vi "FTW-JSON-Core-GetFlattenedValue.vi"(0 "JSON Element":i64 format="%016x", 5 "Element Data Name":string, 7 "LabVIEW Type":T1, 9 "Element Default Value":variant, 11 "error in":errorcluster) -> (4 "Flattened Value":string, 15 "error out":errorcluster)   [LabVIEW 2012]
uses:
  Reflection/FTW-Reflection-Types.ctl
  FTW-JSON-Type.ctl
panel:
  # "Inputs"
  # "Outputs"
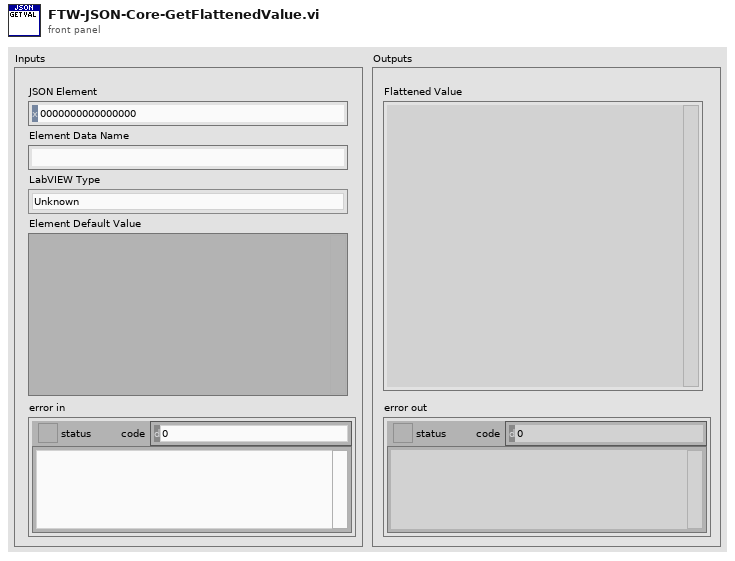
[diagram p1: front panel]
types:
  T1 = typedef "FTW-Reflection-Types.ctl" = enum16{"Unknown", "Void", "Array", "Cluster", "LVObject", "Boolean", "I8", "I16", "I32", "I64", "U8", "U16", "U32", "U64", "SGL", "DBL", "EXT", "CSG", "CDB", "CXT", "FXP", "EnumU8", "EnumU16", "EnumU32", "EnumU64", "SGLwithUnit", "DBLwithUnit", "EXTwithUnit", "CSGwithUnit", "CDBwithUnit", "CXTwithUnit", "String", "Path", "Picture", "Tag", "LVVariant", "Timestamp", "WaveformI8", "WaveformI16", "WaveformI32", "WaveformI64", "WaveformU8", "WaveformU16", "WaveformU32", "WaveformU64", "WaveformSGL", "WaveformDBL", "WaveformEXT", "WaveformCSG", "WaveformCDB", "WaveformCXT", "WaveformDigital", "WaveformUnknownType", "DigitalData", "DynamicData", "ExternalData", "FileByteStream", "TDMStream", "dotNET", "ActiveX", "VIServerReference", "VIReference", "ApplicationInstance", "Menu", "ConnectionDataSocket", "ConnectionVISA", "ConnectionBluetooth", "ConnectionIrDA", "ConnectionTCP", "ConnectionUDP", "ConnectionHTTPClient", "ConnectionFTP", "Occurrence", "Notifier", "Queue", "Rendezvous", "Semaphore", "RTFIFO", "EventPublisher", "EventRegistration", "EventCallback", "DataValueReference", "GenericClass", "GenericClassTag", "GenericClassDeepCopy", "GenericClassFlattened", "GenericClassTagFlattened", "GenericReferenceType", "WindowsRegistry", "OverloadedDatalogRef", "ReferenceUnknownType"}
  T2 = typedef "FTW-JSON-Type.ctl" = enum16{"Object", "Array", "String", "Integer", "Floating Point", "true", "false", "null", "undefined"}
  T3 = cluster{"Element Name":string, "Element Type":T1, "Element Value":variant}[]
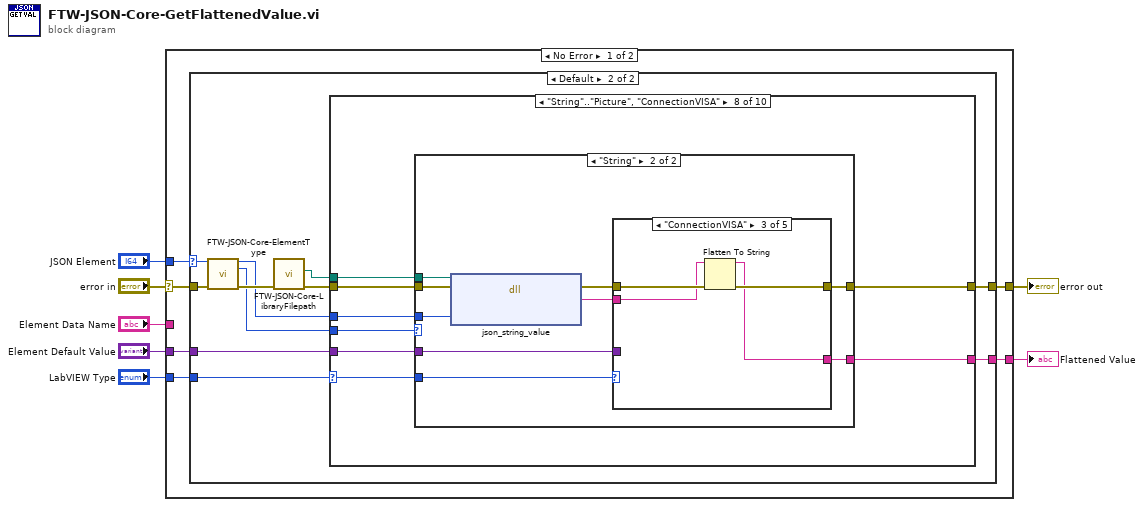
[diagram p0: block diagram]
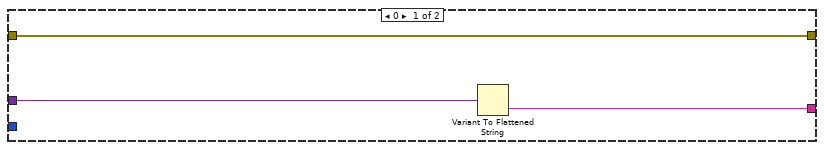
[diagram p2: hidden frame]
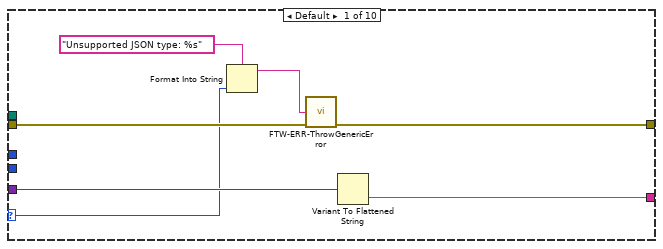
[diagram p3: hidden frame]
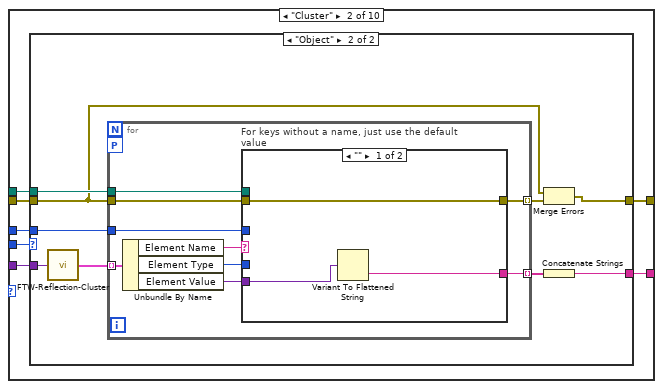
[diagram p4: hidden frame]
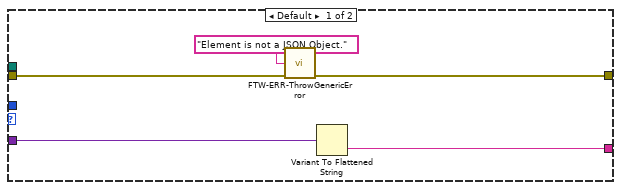
[diagram p5: hidden frame]
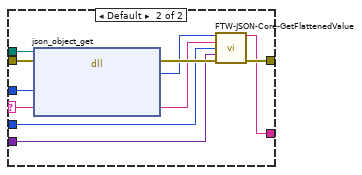
[diagram p6: hidden frame]
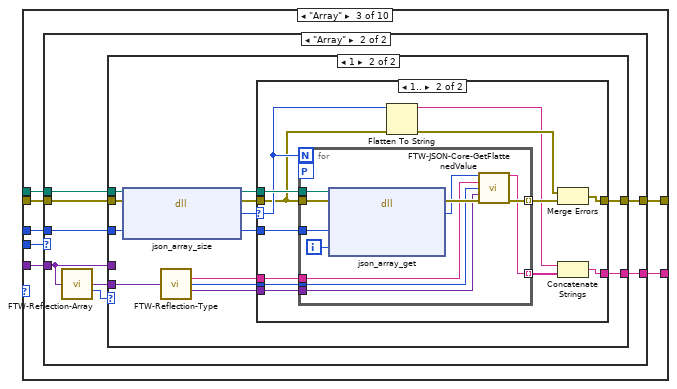
[diagram p7: hidden frame]
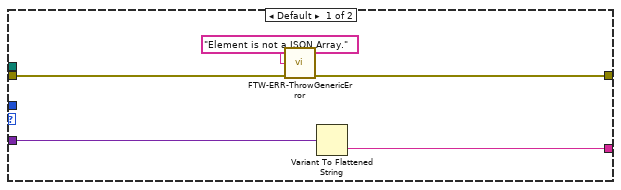
[diagram p8: hidden frame]
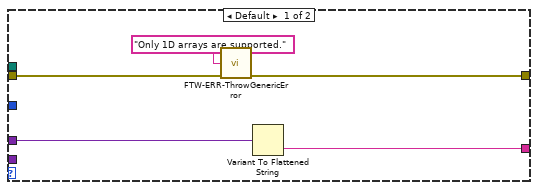
[diagram p9: hidden frame]
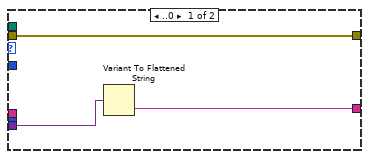
[diagram p10: hidden frame]
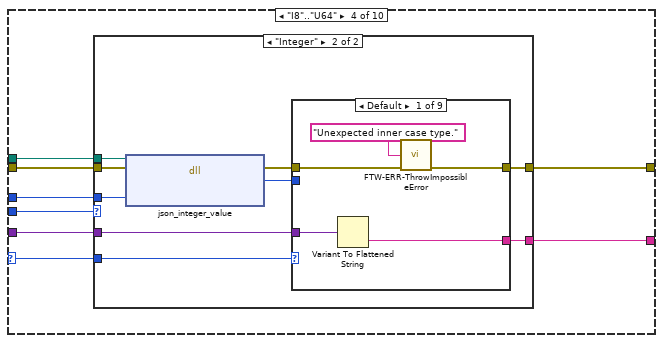
[diagram p11: hidden frame]
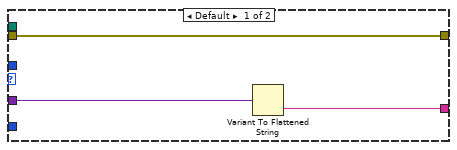
[diagram p12: hidden frame]
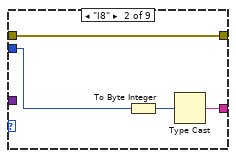
[diagram p13: hidden frame]
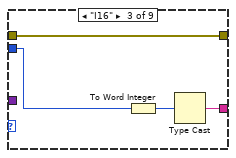
[diagram p14: hidden frame]
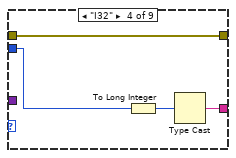
[diagram p15: hidden frame]
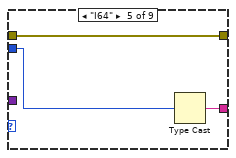
[diagram p16: hidden frame]
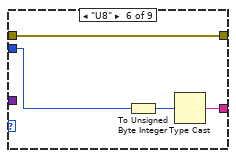
[diagram p17: hidden frame]
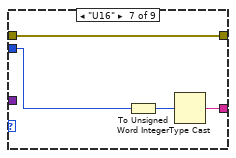
[diagram p18: hidden frame]
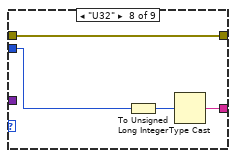
[diagram p19: hidden frame]
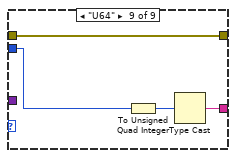
[diagram p20: hidden frame]
diagram:
  n1 = case shown="No Error" "error in" {
    selector: "error in" -> [w9 w424]
    tunnel: [w13 w424] -> w7
    tunnel: "JSON Element" -> [w8 _]
    tunnel: [w12 w422] -> w5
    tunnel: "LabVIEW Type" -> [w11 _]
    tunnel: "Element Default Value" -> [w10 w423]
    tunnel: "Element Data Name" -> [_ _]
    frame No Error {
      n2 = case shown="Default" w8 {
        selector: w8 -> [_ w17]
        tunnel: [w14 w27] -> w13
        tunnel: [w15 w26] -> w12
        tunnel: w11 -> [_ w23]
        tunnel: w10 -> [w16 w22]
        tunnel: w9 -> [w14 w21]
        frame 0 {
          n3 = Variant To Flattened String(Variant=w16) -> (data string=w15:string)  [unwired: 1 out]
        }
        frame Default {
          n4 = call "FTW-JSON-Core-ElementType.vi"("JSON Element"=w17, "error in"=w21) -> ("JSON Element out"=w19:i64, "JSON Type"=w18:T2, "error out"=w20:errorcluster)  [unwired: 11 in]
          n5 = call "FTW-JSON-Core-LibraryFilepath.vi"("error in"=w20) -> ("error out"=w25:errorcluster, "JSON Library Filepath"=w24:path)  [unwired: 9 in]
          n6 = case shown="\"String\"..\"Picture\", \"ConnectionVISA\"" w23 {
            selector: w23 -> [w28 _ _ w147 w203 w286 _ w339 _ _]
            tunnel: [w31 w37 w83 w144 w200 w283 w319 w336 w378 w409] -> w27
            tunnel: [w29 w40 w84 w149 w205 w288 w323 w341 w382 w412] -> w26
            tunnel: w25 -> [w32 w36 w82 w150 w206 w289 w324 w342 w383 w413]
            tunnel: w24 -> [_ w39 w80 w151 w207 w290 w325 w343 w384 _]
            tunnel: w19 -> [_ w38 w79 w146 w202 w285 w321 w338 w380 _]
            tunnel: w22 -> [w30 w41 w85 w148 w204 w287 w322 w340 w381 w411]
            tunnel: w18 -> [_ w35 w81 w145 w201 w284 w320 w337 w379 w410]
            frame Default {
              n7 = Format Into String(format string="Unsupported JSON type: %s", w28) -> (resulting string=w34:string)  [unwired: 2 in, 1 out]
              n8 = call "FTW-ERR-ThrowGenericError.vi"("Error Message"=w34, "error in"=w32) -> ("error out"=w31:errorcluster)  [unwired: 13 in]
              n9 = Variant To Flattened String(Variant=w30) -> (data string=w29:string)  [unwired: 1 out]
            }
            frame "Cluster" {
              n10 = case shown="\"Object\"" w35 {
                tunnel: w41 -> [w44 w54]
                tunnel: [w43 w52] -> w40
                tunnel: w39 -> [_ w51]
                tunnel: w38 -> [_ w49]
                tunnel: [w45 w48] -> w37
                tunnel: w36 -> [w46 w47]
                frame Default {
                  n11 = call "FTW-ERR-ThrowGenericError.vi"("Error Message"="Element is not a JSON Object.", "error in"=w46) -> ("error out"=w45:errorcluster)  [unwired: 13 in]
                  n12 = Variant To Flattened String(Variant=w44) -> (data string=w43:string)  [unwired: 1 out]
                }
                frame "Object" {
                  n13 = call "FTW-Reflection-Cluster.vi"("Cluster"=w54) -> ("Cluster Elements"=w55:T3)  [unwired: 14 in]
                  n14 = for {
                    tunnel: w55 -> [w63] mode=indexing
                    tunnel: [w60] -> w53 mode=indexing
                    tunnel: w51 -> [w57]
                    tunnel: w49 -> [w56]
                    tunnel: w47 -> [w64]
                    tunnel: [w58] -> w50 mode=indexing
                    workers-P: _ -> [_]
                    n15 = Unbundle By Name(w63) -> ("Element Name"=w62:string, "Element Type"=w59:T1, "Element Value"=w61:variant)
                    n16 = case "For keys without a name, just use the default value" shown="\"\"" w62 {
                      selector: w62 -> [_ w74]
                      tunnel: w57 -> [_ w77]
                      tunnel: w64 -> [w65 w76]
                      tunnel: w61 -> [w67 w70]
                      tunnel: [w66 w71] -> w60
                      tunnel: w56 -> [_ w75]
                      tunnel: w59 -> [_ w69]
                      tunnel: [w65 w72] -> w58
                      frame "" {
                        n17 = Variant To Flattened String(Variant=w67) -> (data string=w66:string)  [unwired: 1 out]
                      }
                      frame Default {
                        n18 = dll-call lib="?" fn="json_object_get"(path in=w77, error in=w76, "JSON Object Pointer"=w75, "Element Key"=w74) -> (error out=w78:errorcluster, "JSON Element Pointer"=w73:i64, "Element Key"=w68:string)  [unwired: 2 in, 1 out]
                        n19 = call "FTW-JSON-Core-GetFlattenedValue.vi"("JSON Element"=w73, "Element Data Name"=w68, "LabVIEW Type"=w69, "Element Default Value"=w70, "error in"=w78) -> ("Flattened Value"=w71:string, "error out"=w72:errorcluster)  [unwired: 9 in]
                      }
                    }
                  }
                  n20 = Merge Errors(w47, w50) -> (w48:errorcluster)
                  n21 = Concatenate Strings(w53) -> (w52:string)
                }
              }
            }
            frame "Array" {
              n22 = case shown="\"Array\"" w81 {
                tunnel: w85 -> [w88 w91]
                tunnel: [w87 w98] -> w84
                tunnel: [w86 w97] -> w83
                tunnel: w82 -> [w89 w96]
                tunnel: w80 -> [_ w93]
                tunnel: w79 -> [_ w92]
                frame Default {
                  n23 = call "FTW-ERR-ThrowGenericError.vi"("Error Message"="Element is not a JSON Array.", "error in"=w89) -> ("error out"=w86:errorcluster)  [unwired: 13 in]
                  n24 = Variant To Flattened String(Variant=w88) -> (data string=w87:string)  [unwired: 1 out]
                }
                frame "Array" {
                  n25 = call "FTW-Reflection-Array.vi"("Array"=w91) -> ("Default Array Element"=w95:variant, "Number of Dimensions"=w94:i32)  [unwired: 13 in]
                  n26 = case shown="1" w94 {
                    tunnel: [w100 w116] -> w98
                    tunnel: [w101 w115] -> w97
                    tunnel: w96 -> [w102 w114]
                    tunnel: w95 -> [_ w108]
                    tunnel: w93 -> [_ w113]
                    tunnel: w92 -> [_ w112]
                    tunnel: w91 -> [w99 _]
                    frame Default {
                      n27 = call "FTW-ERR-ThrowGenericError.vi"("Error Message"="Only 1D arrays are supported.", "error in"=w102) -> ("error out"=w101:errorcluster)  [unwired: 13 in]
                      n28 = Variant To Flattened String(Variant=w99) -> (data string=w100:string)  [unwired: 1 out]
                    }
                    frame 1 {
                      n29 = dll-call lib="?" fn="json_array_size"(path in=w113, error in=w114, "Array Pointer"=w112) -> (path out=w111:path, error out=w109:errorcluster, "Array Size"=w105:i32, "Array Pointer"=w110:i64)  [unwired: 1 in]
                      n30 = call "FTW-Reflection-Type.vi"("Anything"=w108) -> ("Data Name"=w104:string, "LabVIEW Type"=w107:T1, "Variant Type and Value"=w106:variant)  [unwired: 12 in]
                      n31 = case shown="1.." w105 {
                        selector: w105 -> [_ w124]
                        tunnel: [w119 w132] -> w116
                        tunnel: [w117 w131] -> w115
                        tunnel: w111 -> [_ w130]
                        tunnel: w110 -> [_ w129]
                        tunnel: w109 -> [w117 w121]
                        tunnel: w107 -> [_ w127]
                        tunnel: w106 -> [w118 w126]
                        tunnel: w104 -> [_ w120]
                        frame ..0 {
                          n32 = Variant To Flattened String(Variant=w118) -> (data string=w119:string)  [unwired: 1 out]
                        }
                        frame 1.. {
                          n33 = for {
                            N: w124 -> [_]
                            tunnel: w130 -> [w142]
                            tunnel: w129 -> [w140]
                            workers-P: _ -> [_]
                            tunnel: w121 -> [w141]
                            tunnel: [w138] -> w128 mode=indexing
                            tunnel: w127 -> [w134]
                            tunnel: w126 -> [w135]
                            tunnel: [w136] -> w125 mode=indexing
                            tunnel: w120 -> [w133]
                            i -> [w139]
                            n34 = dll-call lib="?" fn="json_array_get"(path in=w142, error in=w141, "Array Pointer"=w140, "Index"=w139) -> (error out=w143:errorcluster, "Array Element"=w137:i64)  [unwired: 3 in, 1 out]
                            n35 = call "FTW-JSON-Core-GetFlattenedValue.vi"("JSON Element"=w137, "Element Data Name"=w133, "LabVIEW Type"=w134, "Element Default Value"=w135, "error in"=w143) -> ("Flattened Value"=w136:string, "error out"=w138:errorcluster)  [unwired: 9 in]
                          }
                          n36 = Flatten To String(anything=w124, error in (no error)=w121) -> (data string=w122:string, error out=w123:errorcluster)  [unwired: 2 in, 1 out]
                          n37 = Merge Errors(w123, w128) -> (w131:errorcluster)
                          n38 = Concatenate Strings(w122, w125) -> (w132:string)
                        }
                      }
                    }
                  }
                }
              }
            }
            frame "I8".."U64" {
              n39 = case shown="\"Integer\"" w145 {
                tunnel: w151 -> [_ w163]
                tunnel: w146 -> [_ w162]
                tunnel: w150 -> [w152 w161]
                tunnel: w148 -> [w154 w155]
                tunnel: [w153 w156] -> w149
                tunnel: [w152 w159] -> w144
                tunnel: w147 -> [_ w160]
                frame Default {
                  n40 = Variant To Flattened String(Variant=w154) -> (data string=w153:string)  [unwired: 1 out]
                }
                frame "Integer" {
                  n41 = dll-call lib="?" fn="json_integer_value"(path in=w163, error in=w161, "JSON Element Pointer"=w162) -> (error out=w158:errorcluster, "I64 Value"=w157:i64)  [unwired: 2 in, 1 out]
                  n42 = case shown="Default" w160 {
                    tunnel: [w167 w172 w176 w180 w183 w187 w191 w195 w199] -> w159
                    tunnel: w158 -> [w168 w172 w176 w180 w183 w187 w191 w195 w199]
                    tunnel: w157 -> [_ w170 w174 w178 w181 w185 w189 w193 w197]
                    tunnel: [w164 w171 w175 w179 w182 w186 w190 w194 w198] -> w156
                    tunnel: w155 -> [w165 _ _ _ _ _ _ _ _]
                    frame Default {
                      n43 = Variant To Flattened String(Variant=w165) -> (data string=w164:string)  [unwired: 1 out]
                      n44 = call "FTW-ERR-ThrowImpossibleError.vi"("Reason this error should never happen"="Unexpected inner case type.", "error in"=w168) -> ("error out"=w167:errorcluster)  [unwired: 13 in]
                    }
                    frame "I8" {
                      n45 = To Byte Integer(number=w170) -> (8bit integer=w169:i8)
                      n46 = Type Cast(x=w169) -> (*(type *) &x=w171:string)  [unwired: 1 in]
                    }
                    frame "I16" {
                      n47 = To Word Integer(number=w174) -> (16bit integer=w173:i16)
                      n48 = Type Cast(x=w173) -> (*(type *) &x=w175:string)  [unwired: 1 in]
                    }
                    frame "I32" {
                      n49 = To Long Integer(number=w178) -> (32bit integer=w177:i32)
                      n50 = Type Cast(x=w177) -> (*(type *) &x=w179:string)  [unwired: 1 in]
                    }
                    frame "I64" {
                      n51 = Type Cast(x=w181) -> (*(type *) &x=w182:string)  [unwired: 1 in]
                    }
                    frame "U8" {
                      n52 = To Unsigned Byte Integer(number=w185) -> (unsigned 8bit integer=w184:u8)
                      n53 = Type Cast(x=w184) -> (*(type *) &x=w186:string)  [unwired: 1 in]
                    }
                    frame "U16" {
                      n54 = To Unsigned Word Integer(number=w189) -> (unsigned 16bit integer=w188:u16)
                      n55 = Type Cast(x=w188) -> (*(type *) &x=w190:string)  [unwired: 1 in]
                    }
                    frame "U32" {
                      n56 = To Unsigned Long Integer(number=w193) -> (unsigned 32bit integer=w192:u32)
                      n57 = Type Cast(x=w192) -> (*(type *) &x=w194:string)  [unwired: 1 in]
                    }
                    frame "U64" {
                      n58 = To Unsigned Quad Integer(1:w197) -> (0:w196:u64)
                      n59 = Type Cast(x=w196) -> (*(type *) &x=w198:string)  [unwired: 1 in]
                    }
                  }
                }
              }
            }
            frame "EnumU8".."EnumU64" {
              n60 = case shown="\"Integer\"" w201 {
                tunnel: w207 -> [_ w219 w259]
                tunnel: w202 -> [_ w218 w257]
                tunnel: w206 -> [w208 w217 w258]
                tunnel: w204 -> [w210 w211 w256]
                tunnel: [w209 w212 w253] -> w205
                tunnel: [w208 w215 w254] -> w200
                tunnel: w203 -> [_ w216 w255]
                frame Default {
                  n61 = Variant To Flattened String(Variant=w210) -> (data string=w209:string)  [unwired: 1 out]
                }
                frame "String" {
                  n62 = dll-call lib="?" fn="json_string_value"(path in=w219, error in=w217, "JSON Element Pointer"=w218) -> (error out=w214:errorcluster, "String Value"=w213:string)  [unwired: 2 in, 1 out]
                  n63 = case shown="Default" w216 {
                    tunnel: [w223 w231 w238 w245 w252] -> w215
                    tunnel: w214 -> [w224 w231 w238 w245 w252]
                    tunnel: w213 -> [_ w228 w235 w242 w249]
                    tunnel: [w220 w227 w234 w241 w248] -> w212
                    tunnel: w211 -> [w221 w230 w237 w244 w251]
                    frame Default {
                      n64 = Variant To Flattened String(Variant=w221) -> (data string=w220:string)  [unwired: 1 out]
                      n65 = call "FTW-ERR-ThrowImpossibleError.vi"("Reason this error should never happen"="Unexpected inner case type.", "error in"=w224) -> ("error out"=w223:errorcluster)  [unwired: 13 in]
                    }
                    frame "EnumU8" {
                      n66 = call "FTW-Reflection-Enum.vi"("Enum"=w230) -> ("Enum Items"=w229:string[])  [unwired: 12 in, 2 out]
                      n67 = Search 1D Array(1D array=w229, element=w228) -> (index of element=w226:i32)  [unwired: 1 in]
                      n68 = To Unsigned Byte Integer(number=w226) -> (unsigned 8bit integer=w225:u8)
                      n69 = Type Cast(x=w225) -> (*(type *) &x=w227:string)  [unwired: 1 in]
                    }
                    frame "EnumU16" {
                      n70 = call "FTW-Reflection-Enum.vi"("Enum"=w237) -> ("Enum Items"=w236:string[])  [unwired: 12 in, 2 out]
                      n71 = Search 1D Array(1D array=w236, element=w235) -> (index of element=w233:i32)  [unwired: 1 in]
                      n72 = To Unsigned Word Integer(number=w233) -> (unsigned 16bit integer=w232:u16)
                      n73 = Type Cast(x=w232) -> (*(type *) &x=w234:string)  [unwired: 1 in]
                    }
                    frame "EnumU32" {
                      n74 = call "FTW-Reflection-Enum.vi"("Enum"=w244) -> ("Enum Items"=w243:string[])  [unwired: 12 in, 2 out]
                      n75 = Search 1D Array(1D array=w243, element=w242) -> (index of element=w240:i32)  [unwired: 1 in]
                      n76 = To Unsigned Long Integer(number=w240) -> (unsigned 32bit integer=w239:u32)
                      n77 = Type Cast(x=w239) -> (*(type *) &x=w241:string)  [unwired: 1 in]
                    }
                    frame "EnumU64" {
                      n78 = call "FTW-Reflection-Enum.vi"("Enum"=w251) -> ("Enum Items"=w250:string[])  [unwired: 12 in, 2 out]
                      n79 = Search 1D Array(1D array=w250, element=w249) -> (index of element=w247:i32)  [unwired: 1 in]
                      n80 = To Unsigned Quad Integer(1:w247) -> (0:w246:u64)
                      n81 = Type Cast(x=w246) -> (*(type *) &x=w248:string)  [unwired: 1 in]
                    }
                  }
                }
                frame "Integer" {
                  n82 = dll-call lib="?" fn="json_integer_value"(path in=w259, error in=w258, "JSON Element Pointer"=w257) -> (error out=w261:errorcluster, "I64 Value"=w260:i64)  [unwired: 2 in, 1 out]
                  n83 = case shown="Default" w255 {
                    tunnel: [w265 w270 w274 w278 w282] -> w254
                    tunnel: w261 -> [w266 w270 w274 w278 w282]
                    tunnel: w260 -> [_ w268 w272 w276 w280]
                    tunnel: [w262 w269 w273 w277 w281] -> w253
                    tunnel: w256 -> [w263 _ _ _ _]
                    frame Default {
                      n84 = Variant To Flattened String(Variant=w263) -> (data string=w262:string)  [unwired: 1 out]
                      n85 = call "FTW-ERR-ThrowImpossibleError.vi"("Reason this error should never happen"="Unexpected inner case type.", "error in"=w266) -> ("error out"=w265:errorcluster)  [unwired: 13 in]
                    }
                    frame "EnumU8" {
                      n86 = To Unsigned Byte Integer(number=w268) -> (unsigned 8bit integer=w267:u8)
                      n87 = Type Cast(x=w267) -> (*(type *) &x=w269:string)  [unwired: 1 in]
                    }
                    frame "EnumU16" {
                      n88 = To Unsigned Word Integer(number=w272) -> (unsigned 16bit integer=w271:u16)
                      n89 = Type Cast(x=w271) -> (*(type *) &x=w273:string)  [unwired: 1 in]
                    }
                    frame "EnumU32" {
                      n90 = To Unsigned Long Integer(number=w276) -> (unsigned 32bit integer=w275:u32)
                      n91 = Type Cast(x=w275) -> (*(type *) &x=w277:string)  [unwired: 1 in]
                    }
                    frame "EnumU64" {
                      n92 = To Unsigned Quad Integer(1:w280) -> (0:w279:u64)
                      n93 = Type Cast(x=w279) -> (*(type *) &x=w281:string)  [unwired: 1 in]
                    }
                  }
                }
              }
            }
            frame "SGL".."EXT" {
              n94 = case shown="\"Integer\", \"Floating Point\"" w284 {
                tunnel: w290 -> [_ w302]
                tunnel: w285 -> [_ w301]
                tunnel: w289 -> [w291 w300]
                tunnel: w287 -> [w293 w294]
                tunnel: [w292 w295] -> w288
                tunnel: [w291 w298] -> w283
                tunnel: w286 -> [_ w299]
                frame Default {
                  n95 = Variant To Flattened String(Variant=w293) -> (data string=w292:string)  [unwired: 1 out]
                }
                frame "Integer", "Floating Point" {
                  n96 = dll-call lib="?" fn="json_number_value"(path in=w302, error in=w300, "JSON Element Pointer"=w301) -> (error out=w297:errorcluster, "DBL Value"=w296:dbl)  [unwired: 2 in, 1 out]
                  n97 = case shown="Default" w299 {
                    tunnel: [w306 w311 w314 w318] -> w298
                    tunnel: w297 -> [w307 w311 w314 w318]
                    tunnel: w296 -> [_ w308 w312 w316]
                    tunnel: [w303 w310 w313 w317] -> w295
                    tunnel: w294 -> [w304 _ _ _]
                    frame Default {
                      n98 = Variant To Flattened String(Variant=w304) -> (data string=w303:string)  [unwired: 1 out]
                      n99 = call "FTW-ERR-ThrowImpossibleError.vi"("Reason this error should never happen"="Unexpected inner case type.", "error in"=w307) -> ("error out"=w306:errorcluster)  [unwired: 13 in]
                    }
                    frame "SGL" {
                      n100 = To Single Precision Float(number=w308) -> (single precision float=w309:sgl)
                      n101 = Type Cast(x=w309) -> (*(type *) &x=w310:string)  [unwired: 1 in]
                    }
                    frame "DBL" {
                      n102 = Type Cast(x=w312) -> (*(type *) &x=w313:string)  [unwired: 1 in]
                    }
                    frame "EXT" {
                      n103 = To Extended Precision Float(1:w316) -> (0:w315:ext)
                      n104 = Type Cast(x=w315) -> (*(type *) &x=w317:string)  [unwired: 1 in]
                    }
                  }
                }
              }
            }
            frame "Timestamp" {
              n105 = case shown="Default" w320 {
                tunnel: w325 -> [_ w335]
                tunnel: w321 -> [_ w334]
                tunnel: w324 -> [w326 w333]
                tunnel: w322 -> [w328 _]
                tunnel: [w327 w331] -> w323
                tunnel: [w326 w332] -> w319
                frame Default {
                  n106 = Variant To Flattened String(Variant=w328) -> (data string=w327:string)  [unwired: 1 out]
                }
                frame "Floating Point" {
                  n107 = dll-call lib="?" fn="json_number_value"(path in=w335, error in=w333, "JSON Element Pointer"=w334) -> (error out=w332:errorcluster, "DBL Value"=w330:dbl)  [unwired: 2 in, 1 out]
                  n108 = To Time Stamp(1:w330) -> (0:w329:timestamp)
                  n109 = Type Cast(x=w329) -> (*(type *) &x=w331:string)  [unwired: 1 in]
                }
              }
            }
            frame "String".."Picture", "ConnectionVISA" {
              n110 = case shown="\"String\"" w337 {
                tunnel: w343 -> [_ w355]
                tunnel: w338 -> [_ w354]
                tunnel: w342 -> [w344 w353]
                tunnel: w340 -> [w346 w347]
                tunnel: [w345 w348] -> w341
                tunnel: [w344 w351] -> w336
                tunnel: w339 -> [_ w352]
                frame Default {
                  n111 = Variant To Flattened String(Variant=w346) -> (data string=w345:string)  [unwired: 1 out]
                }
                frame "String" {
                  n112 = dll-call lib="?" fn="json_string_value"(path in=w355, error in=w353, "JSON Element Pointer"=w354) -> (error out=w350:errorcluster, "String Value"=w349:string)  [unwired: 2 in, 1 out]
                  n113 = case shown="\"ConnectionVISA\"" w352 {
                    tunnel: [w359 w363 w367 w372 w377] -> w351
                    tunnel: w350 -> [w360 w364 w368 w373 w377]
                    tunnel: w349 -> [_ w362 w366 w371 w376]
                    tunnel: [w356 w361 w365 w370 w375] -> w348
                    tunnel: w347 -> [w357 _ _ _ _]
                    frame Default {
                      n114 = Variant To Flattened String(Variant=w357) -> (data string=w356:string)  [unwired: 1 out]
                      n115 = call "FTW-ERR-ThrowImpossibleError.vi"("Reason this error should never happen"="Unexpected inner case type.", "error in"=w360) -> ("error out"=w359:errorcluster)  [unwired: 13 in]
                    }
                    frame "String" {
                      n116 = Flatten To String(anything=w362, error in (no error)=w364) -> (data string=w361:string, error out=w363:errorcluster)  [unwired: 2 in, 1 out]
                    }
                    frame "ConnectionVISA" {
                      n117 = Flatten To String(anything=w366, error in (no error)=w368) -> (data string=w365:string, error out=w367:errorcluster)  [unwired: 2 in, 1 out]
                    }
                    frame "Path" {
                      n118 = String To Path(string=w371) -> (path=w369:path)
                      n119 = Flatten To String(anything=w369, error in (no error)=w373) -> (data string=w370:string, error out=w372:errorcluster)  [unwired: 2 in, 1 out]
                    }
                    frame "Picture" {
                      n120 = call "FTW-STR-Encode-Base64.vi"("Input"=w376, "Direction"=enum16{"Encode", "Decode"}."Decode") -> ("Output"=w375:string)
                    }
                  }
                }
              }
            }
            frame "FileByteStream".."ConnectionDataSocket", "ConnectionBluetooth".."ReferenceUnknownType" {
              n121 = case shown="\"String\"" w379 {
                tunnel: w384 -> [_ w399]
                tunnel: w380 -> [_ w398]
                tunnel: w383 -> [w385 w397]
                tunnel: w381 -> [w387 w392]
                tunnel: [w386 w394] -> w382
                tunnel: [w385 w390] -> w378
                frame Default {
                  n122 = Variant To Flattened String(Variant=w387) -> (data string=w386:string)  [unwired: 1 out]
                }
                frame "String" {
                  w395 = "0x%16x"  # Reference Format
                  n123 = dll-call lib="?" fn="json_string_value"(path in=w399, error in=w397, "JSON Element Pointer"=w398) -> (error out=w389:errorcluster, "String Value"=w396:string, "JSON Element Pointer"=w388:i64)  [unwired: 1 in, 1 out]
                  n124 = Scan From String(format string=w395, input string=w396, error in=w389, default 1=w388) -> (error out=w391:errorcluster, output 1=w393:i64)  [unwired: 1 in, 2 out]
                  n125 = case shown="No Error" w391 {
                    selector: w391 -> [w400 _]
                    tunnel: [w404 w407] -> w394
                    tunnel: w393 -> [w403 _]
                    tunnel: w392 -> [_ w408]
                    tunnel: [w400 w406] -> w390
                    frame No Error {
                      n126 = Type Cast(type=refnum<k0> refnum, x=w403) -> (*(type *) &x=w402:refnum<k0>)
                      n127 = Type Cast(x=w402) -> (*(type *) &x=w404:string)  [unwired: 1 in]
                    }
                    frame Error {
                      n128 = Variant To Flattened String(Variant=w408) -> (data string=w407:string)  [unwired: 1 out]
                      n129 = call "FTW-ERR-ThrowGenericError.vi"("Error Message"="Unexpected reference format.") -> ("error out"=w406:errorcluster)  [unwired: 14 in]
                    }
                  }
                }
              }
            }
            frame "Boolean" {
              n130 = case shown="Default" w410 {
                selector: w410 -> [_ w419]
                tunnel: w413 -> [w414 w420]
                tunnel: w411 -> [w416 _]
                tunnel: [w415 w421] -> w412
                tunnel: [w414 w420] -> w409
                frame Default {
                  n131 = Variant To Flattened String(Variant=w416) -> (data string=w415:string)  [unwired: 1 out]
                }
                frame "true", "false" {
                  n132 = Equal?(x=w419, y=FTW-JSON-Type."true" ("x")) -> (x = y?=w417:bool)
                  n133 = Type Cast(x=w417) -> (*(type *) &x=w421:string)  [unwired: 1 in]
                }
              }
            }
          }
        }
      }
    }
    frame Error {
      n134 = Variant To Flattened String(Variant=w423) -> (data string=w422:string)  [unwired: 1 out]
    }
  }
  "error out" <- w7
  "Flattened Value" <- w5
